vi "Read (Single Point).vi"(8 "error in (no error)":errorcluster, 11 "VISA resource name":refnum<visa-resource-name>) -> (0 "error out":errorcluster, 2 "Measurement":dbl format="%#_8f", 3 "VISA resource name out":refnum<visa-resource-name>)   [LabVIEW 2024, in "U1250 Series Digital Multimeter.lvlib"]
doc: "Reads and returns a single measurement from the instrument."
uses:
  U1250 Series Digital Multimeter.lvlib
panel:
  out "read buffer":string
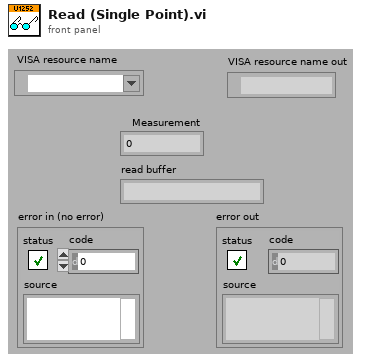
[diagram p1: front panel]
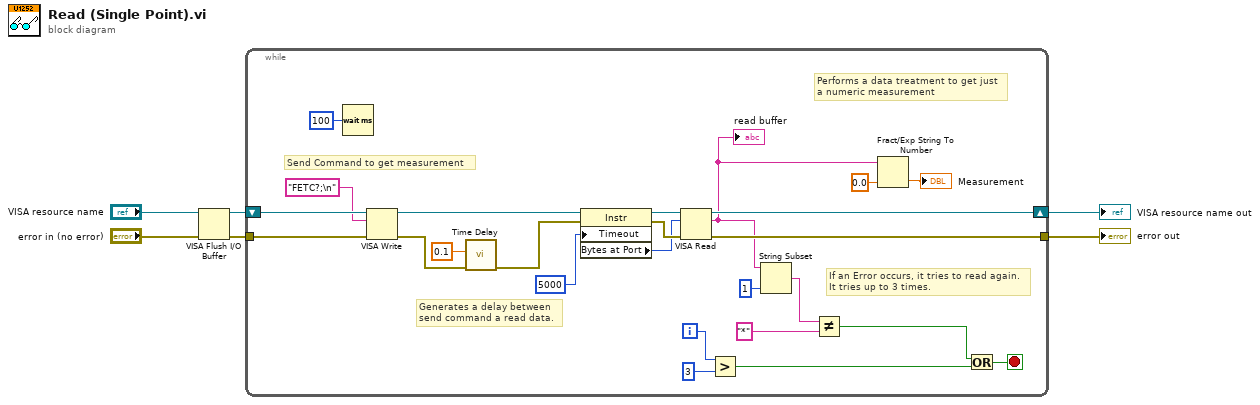
[diagram p0: block diagram]
diagram:
  n1 = VISA Flush I/O Buffer(VISA resource name="VISA resource name", error in (no error)="error in (no error)") -> (VISA resource name out=w3:refnum<visa-resource-name>, error out=w4:errorcluster)  [unwired: 1 in]
  n2 = while {
    shift-right: [w30] -> w5
    shift-left: w3 -> [w31]
    tunnel: w4 -> [w22]
    tunnel: [w19] -> w6
    i -> [w24]
    stop <- w11 stop-if-true
    # "If an Error occurs, it tries to read again.\nIt tries up to 3 times."
    # "Generates a delay between\nsend command a read data."
    # "Performs a data treatment to get just\na numeric measurement"
    # "Send Command to get measurement"
    n3 = Wait (ms)(milliseconds to wait=u32 100) -> ()  [unwired: 1 out]
    n4 = VISA Write(VISA resource name=w31, write buffer="FETC?;\n", error in (no error)=w22) -> (VISA resource name out=w28:refnum<visa-resource-name>, error out=w14:errorcluster)  [unwired: 1 out]
    n5 = call "Time Delay"("error in (no error)"=w14, "Delay Time (s)"=0.1) -> ("error out"=w13:errorcluster)  [unwired: 9 in]
    n6 = property class="Instr"(reference=w28, error in=w13, "Timeout"=u32 5000 ("General Settings:Timeout Value")) -> (reference out=w26:refnum<visa-resource-name>, error out=w25:errorcluster, "Bytes at Port"=w16:u32)
    n7 = VISA Read(VISA resource name=w26, byte count=w16, error in (no error)=w25) -> (VISA resource name out=w30:refnum<visa-resource-name>, read buffer=w7:string, error out=w19:errorcluster)  [unwired: 1 out]
    "read buffer" <- w7
    n8 = Greater?(x=w24, y=3) -> (0:w10:bool)
    n9 = String Subset(string=w7, length (rest)=1 ("length (rest)")) -> (substring=w17:string)  [unwired: 1 in]
    n10 = Not Equal?(x=w17, y="*") -> (x != y?=w12:bool)
    n11 = Fract/Exp String To Number(string=w7, default (0 dbl)=0.0 ("default (0 DBL)")) -> (number=→"Measurement":dbl)  [unwired: 2 in, 1 out]
    n12 = Or(x=w12, y=w10) -> (x .or. y?=w11:bool)
  }
  "error out" <- w6
  "VISA resource name out" <- w5
